vi "stop daemon.vi"(8 "error in (no error)":errorcluster) -> (0 "error out":errorcluster)   [LabVIEW 2016, in "update.lvlib"]
uses:
  update.lvlib
panel:
  out "standard error":string caption="标准错误"
  out "standard output":string caption="标准输出"
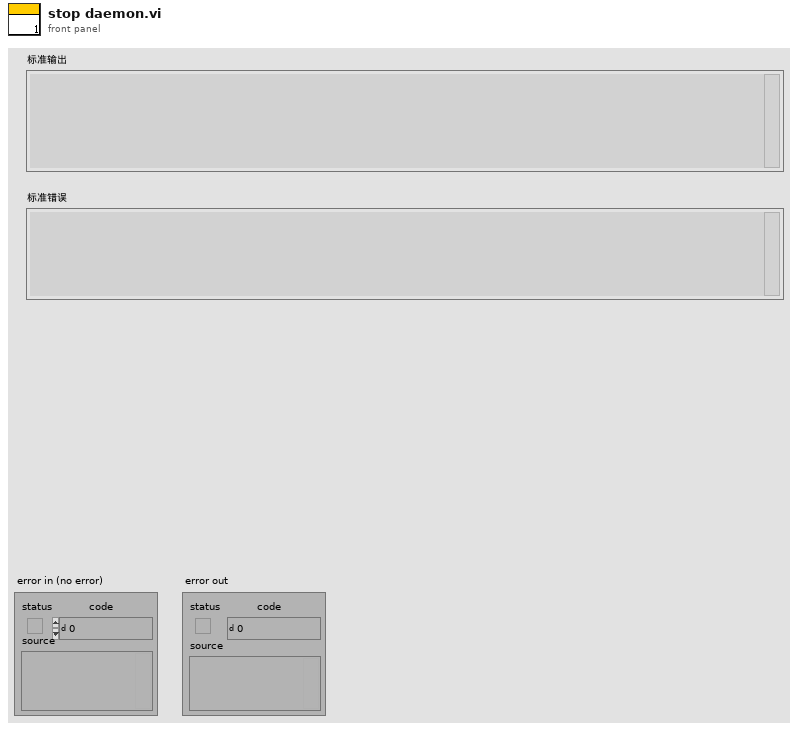
[diagram p1: front panel]
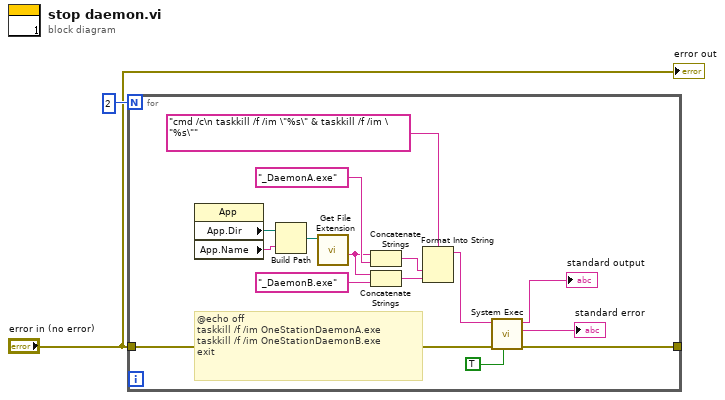
[diagram p0: block diagram]
diagram:
  n1 = for {
    N: 2 -> [_]
    tunnel: "error in (no error)" -> [w7]
    tunnel: [w8] -> _
    # "@echo off\ntaskkill /f /im OneStationDaemonA.exe\ntaskkill /f /im OneStationDaemonB.exe\nexit"
    n2 = property class="App"() -> ("App.Dir"=w5:path, "App.Name"=w4:string)  [unwired: 2 in, 2 out]
    n3 = Build Path(base path=w5, name or relative path=w4) -> (appended path=w3:path)
    n4 = call <vilib>:"Get File Extension.vi"("file"=w3) -> ("filename without extension"=w14:string)  [unwired: 6 in, 4 out]
    n5 = Concatenate Strings(w14, "_DaemonA.exe" ("名称或相对路径")) -> (w13:string)
    n6 = Concatenate Strings(w14, "_DaemonB.exe" ("名称或相对路径")) -> (w12:string)
    n7 = Format Into String(format string="cmd /c\n taskkill /f /im \"%s\" & taskkill /f /im \"%s\"" ("格式字符串"), w13, w12) -> (resulting string=w11:string)  [unwired: 2 in, 1 out]
    n8 = call <vilib>:"System Exec.vi"("run minimized? (F)"=TRUE, "error in (no error)"=w7, "command line"=w11) -> ("error out"=w8:errorcluster, "standard error"=→"standard error":string, "standard output"=→"standard output":string)  [unwired: 5 in, 1 out]
  }
  "error out" <- "error in (no error)"
